vi "Init.vi"(8 "Error In":errorcluster, 10 "Folder Path":path, 11 "Plugin Framework In":refnum<class "Measurement Interface.lvclass">) -> (0 "Error Out":errorcluster, 3 "Measurement Interface out":refnum<class "Measurement Interface.lvclass">)   [LabVIEW 2016, in "Measurement Interface.lvlib" / "Measurement Interface.lvclass"]
uses:
  Measurement Interface.lvclass
  Plugins/FPF.lvlibp/Factory Plugin Framework.lvclass
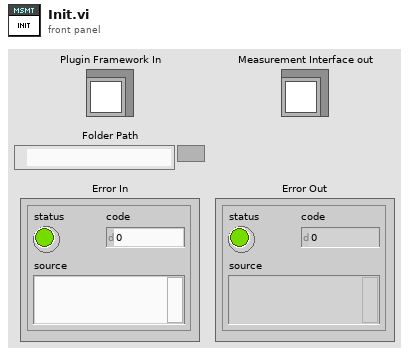
[diagram p1: front panel]
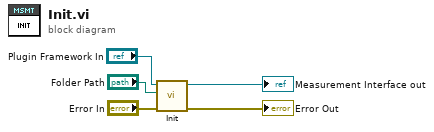
[diagram p0: block diagram]
diagram:
  n1 = call-parent "Init.vi"("Error In"="Error In", "Folder Path"="Folder Path", "Plugin Framework In"="Plugin Framework In") -> ("Error Out"=→"Error Out":errorcluster, "Factory Plugin Framework out"=→"Measurement Interface out":refnum<class "Measurement Interface.lvclass">)  [unwired: 7 in]
